vi "Destroy_Logger.vi"(8 "error in (no error)":errorcluster, 11 "RQMHLogger in":refnum<class "Logger.lvclass">) -> (0 "error out":errorcluster)   [LabVIEW 2024, in "Logger.lvclass"]
uses:
  Logger.lvclass
  Logger.lvclass/Logger.ctl
  HandleHolder/HandleHolder.lvclass/HandleHolder.ctl
  HandleHolder/Read Handle.vi
  LogHandle/Interface/LoggingHandle.lvclass
  HandleHolder/HandleHolder.lvclass
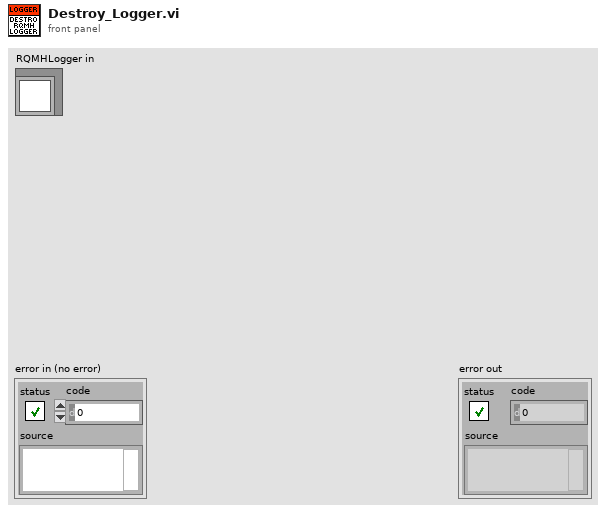
[diagram p1: front panel]
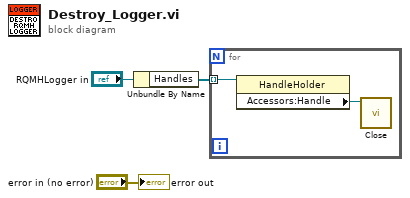
[diagram p0: block diagram]
diagram:
  n1 = Unbundle By Name("RQMHLogger in") -> ("Handles"=w1:refnum<class "HandleHolder.lvclass">[])
  n2 = for {
    tunnel: w1 -> [w5] mode=indexing
    n3 = property class="HandleHolder"(reference=w5) -> ("Accessors:Handle"=w4:refnum<class "LoggingHandle.lvclass">)  [unwired: 1 in, 2 out]
    n4 = call-dynamic "Close.vi"("LoggingHandle in"=w4) -> ()  [unwired: 10 in, 1 out]
  }
  "error out" <- "error in (no error)"
